vi "Update Menu Items.vi"(7 "Device Ref in":T1 format="%.0x", 8 "error in (no error)":errorcluster, 9 "Coords":T2, 10 "MenuRef":refnum<k9>, 11 "Table in":refnum<vi>) -> (0 "error out":errorcluster)   [LabVIEW 2014, in "SLSC configuration System Explorer.lvlib"]
uses:
  SLSC configuration System Explorer.lvlib
  <vilib>/Utility/miscctls.llb/LVPoint32TypeDef.ctl
  <vilib>/NI Veristand/Custom Device API/Custom Device Item Ref.ctl
  Shared/Constants.vi
  <vilib>/NI Veristand/Custom Device API/Get Item Property (U16).vi
  <vilib>/NI Veristand/Custom Device Tools/Custom Device Utility Library/NI VeriStand - Search for Item by Name.vi
  <vilib>/NI Veristand/Custom Device Tools/Custom Device Utility Library/Custom Device Utility Library.lvlib
  <vilib>/NI Veristand/Custom Device API/Custom Device API.lvlib
  Shared/SLSC configuration Shared.lvlib
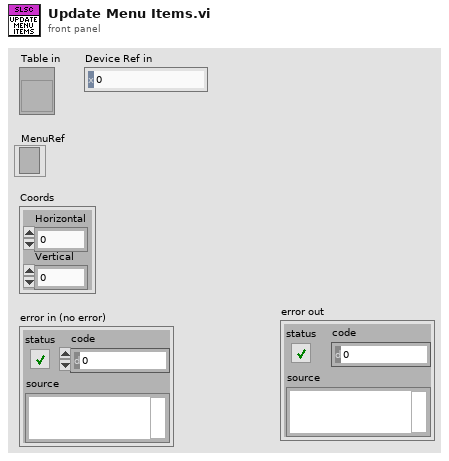
[diagram p1: front panel]
types:
  T1 = typedef "Custom Device API.lvlib/Custom Device Item Ref.ctl" = u64
  T2 = typedef "LVPoint32TypeDef.ctl" = cluster{"Horizontal":i32, "Vertical":i32}
  T3 = typedef "LVRowAndColumnTypeDef.ctl" = cluster{"Row":i32, "Column":i32}
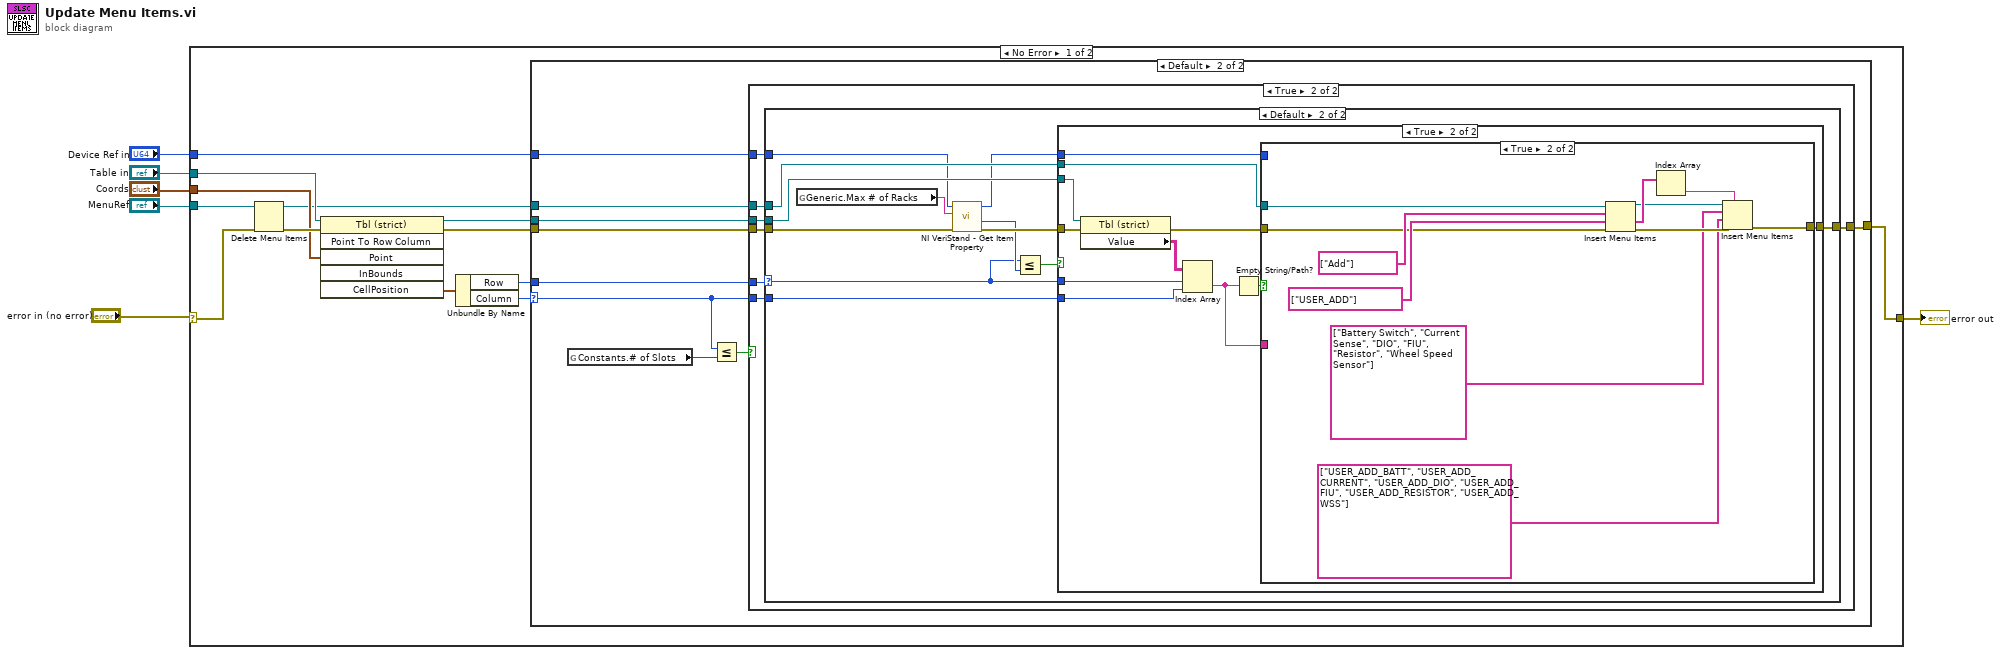
[diagram p0: block diagram]
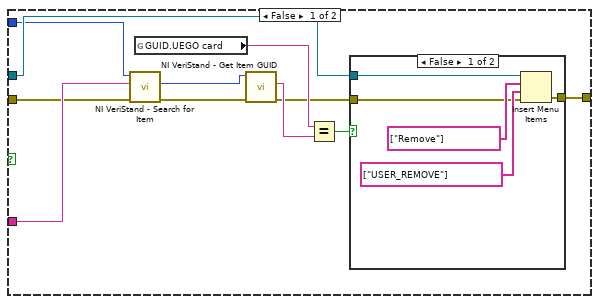
[diagram p6: hidden frame]
diagram:
  n1 = case shown="No Error" "error in (no error)" {
    selector: "error in (no error)" -> [w8 w91]
    tunnel: "MenuRef" -> [w18 _]
    tunnel: "Coords" -> [w17 _]
    tunnel: "Table in" -> [w16 _]
    tunnel: [w9 w91] -> w3
    tunnel: "Device Ref in" -> [w7 _]
    frame No Error {
      n2 = Delete Menu Items(6:w8, 9:w18) -> (0:w19:errorcluster, 3:w12:refnum<k9>)  [unwired: 2 in]
      n3 = invoke class="Tbl (strict)" method="Point To Row Column"(reference=w16, error in=w19, "Point"=w17) -> (reference out=w10:refnum<vi>, error out=w11:errorcluster, "CellPosition"=w15:T3)  [unwired: 3 in, 3 out]
      n4 = Unbundle By Name(w15) -> ("Row"=w13:i32, "Column"=w14:i32)
      n5 = case shown="Default" w14 {
        selector: w14 -> [_ w23]
        tunnel: w13 -> [_ w29]
        tunnel: w12 -> [_ w28]
        tunnel: w11 -> [w20 w27]
        tunnel: w10 -> [_ w26]
        tunnel: [w20 w25] -> w9
        tunnel: w7 -> [_ w24]
        frame 0, 1 {
          # "No menu items for columns 0 and 1"
        }
        frame Default {
          n6 = global read "Constants.vi" "Constants.# of Slots"() -> (w22:u8)
          n7 = Less Or Equal?(x=w23, y=w22) -> (x <= y?=w21:bool)
          n8 = case shown="True" w21 {
            tunnel: w29 -> [_ w37]
            tunnel: w28 -> [_ w36]
            tunnel: w27 -> [w30 w35]
            tunnel: w26 -> [_ w34]
            tunnel: [w30 w33] -> w25
            tunnel: w24 -> [_ w32]
            tunnel: w23 -> [_ w31]
            frame False {
            }
            frame True {
              n9 = case shown="Default" w37 {
                selector: w37 -> [_ w39]
                tunnel: w36 -> [_ w50]
                tunnel: w35 -> [w38 w45]
                tunnel: w34 -> [_ w49]
                tunnel: w31 -> [_ w48]
                tunnel: [w38 w47] -> w33
                tunnel: w32 -> [_ w44]
                frame 0 {
                  # "No menu items for row 0"
                }
                frame Default {
                  n10 = global read "Constants.vi" "Generic.Max # of Racks"() -> (w46:string)
                  n11 = call-poly <vilib>:"NI VeriStand - Get Item Property.vi"("error in (no error)"=w45, "Property Name"=w46, "Item Ref in"=w44) -> ("error out"=w42:errorcluster, "Value"=w40:u16, "Item Ref out"=w43:T1)  [unwired: 5 in, 1 out]
                  n12 = Less Or Equal?(x=w39, y=w40) -> (x <= y?=w41:bool)
                  n13 = case shown="True" w41 {
                    tunnel: w50 -> [_ w62]
                    tunnel: w49 -> [_ w61]
                    tunnel: w48 -> [_ w59]
                    tunnel: [w51 w56] -> w47
                    tunnel: w43 -> [_ w54]
                    tunnel: w42 -> [w51 w53]
                    tunnel: w39 -> [_ w52]
                    frame False {
                      # "User selected outside of the table"
                    }
                    frame True {
                      n14 = property class="Tbl (strict)"(reference=w61, error in=w53) -> (error out=w57:errorcluster, "Value"=w60:string[][])  [unwired: 1 out]
                      n15 = Index Array(array=w60, index (row)=w52, index (col)=w59) -> (element=w55:string)
                      n16 = Empty String/Path?(string/path=w55) -> (empty?=w58:bool)
                      n17 = case shown="True" w58 {
                        tunnel: w62 -> [w73 w90]
                        tunnel: w57 -> [w68 w81]
                        tunnel: [w72 w84] -> w56
                        tunnel: w55 -> [w71 _]
                        tunnel: w54 -> [w63 _]
                        frame False {
                          n18 = call-poly <vilib>:"NI VeriStand - Search for Item.vi"("error in"=w68, "Item Name"=w71, "Section Ref in"=w63) -> ("error out"=w70:errorcluster, "Item Ref"=w69:T1)  [unwired: 5 in, 2 out]
                          n19 = global read "Constants.vi" "GUID.UEGO card"() -> (w66:string)
                          n20 = call <vilib>:"NI VeriStand - Get Item GUID.vi"("error in (no error)"=w70, "Item Ref in"=w69) -> ("error out"=w64:errorcluster, "GUID"=w67:string)  [unwired: 7 in, 1 out]
                          n21 = Equal?(x=w66, y=w67) -> (x = y?=w65:bool)
                          n22 = case shown="False" w65 {
                            tunnel: w73 -> [w77 _]
                            tunnel: [w75 w79] -> w72
                            tunnel: w64 -> [w74 w79]
                            frame False {
                              n23 = Insert Menu Items(6:w74, 7:string[] ["USER_REMOVE"] ("item names"), 8:string[] ["Remove"] ("item names"), 9:w77) -> (0:w75:errorcluster)  [unwired: 2 in, 2 out]
                            }
                            frame True {
                            }
                          }
                        }
                        frame True {
                          n24 = Insert Menu Items(6:w81, 7:string[] ["USER_ADD"] ("item tags"), 8:string[] ["Add"] ("item names"), 9:w90) -> (0:w88:errorcluster, 1:w89:string[], 3:w87:refnum<k9>)  [unwired: 2 in]
                          n25 = Index Array(array=w89) -> (element=w86:string)  [unwired: 1 in]
                          n26 = Insert Menu Items(5:w86, 6:w88, 7:string[] ["USER_ADD_BATT", "USER_ADD_CURRENT", "USER_ADD_DIO", "USER_ADD_FIU", "USER_ADD_RESISTOR", "USER_ADD_WSS"] ("item tags"), 8:string[] ["Battery Switch", "Current Sense", "DIO", "FIU", "Resistor", "Wheel Speed Sensor"] ("item names"), 9:w87) -> (0:w84:errorcluster)  [unwired: 1 in, 2 out]
                        }
                      }
                    }
                  }
                }
              }
            }
          }
        }
      }
    }
    frame Error {
    }
  }
  "error out" <- w3
